vi "Measure P2.vi"(0 "Image Dup In":T1, 11 "Error In":errorcluster) -> (4 "Image Out":T1, 12 "Calibrated Results (P2 Hole)":sgl, 13 "Calibrated Results (P2 Left Edge Angles)":sgl, 14 "Calibrated Results (P2 Right Edge Angle)":sgl, 15 "Error Out":errorcluster)   [LabVIEW 2020, in "BilGör.lvlib"]
uses:
  <vilib>/vision/Image Controls.llb/IMAQ Image.ctl
  <vilib>/vision/Image Controls.llb/Vision Info Type2.ctl
  <vilib>/vision/Measure.llb/Edge Options.ctl
  <vilib>/vision/Measure.llb/Edge Polarity.ctl
  <vilib>/vision/Measure.llb/Straight Edge Options.ctl
  <vilib>/vision/Measure.llb/Straight Edge Process.ctl
  <vilib>/vision/NI_Vision_Development_Module.lvlib
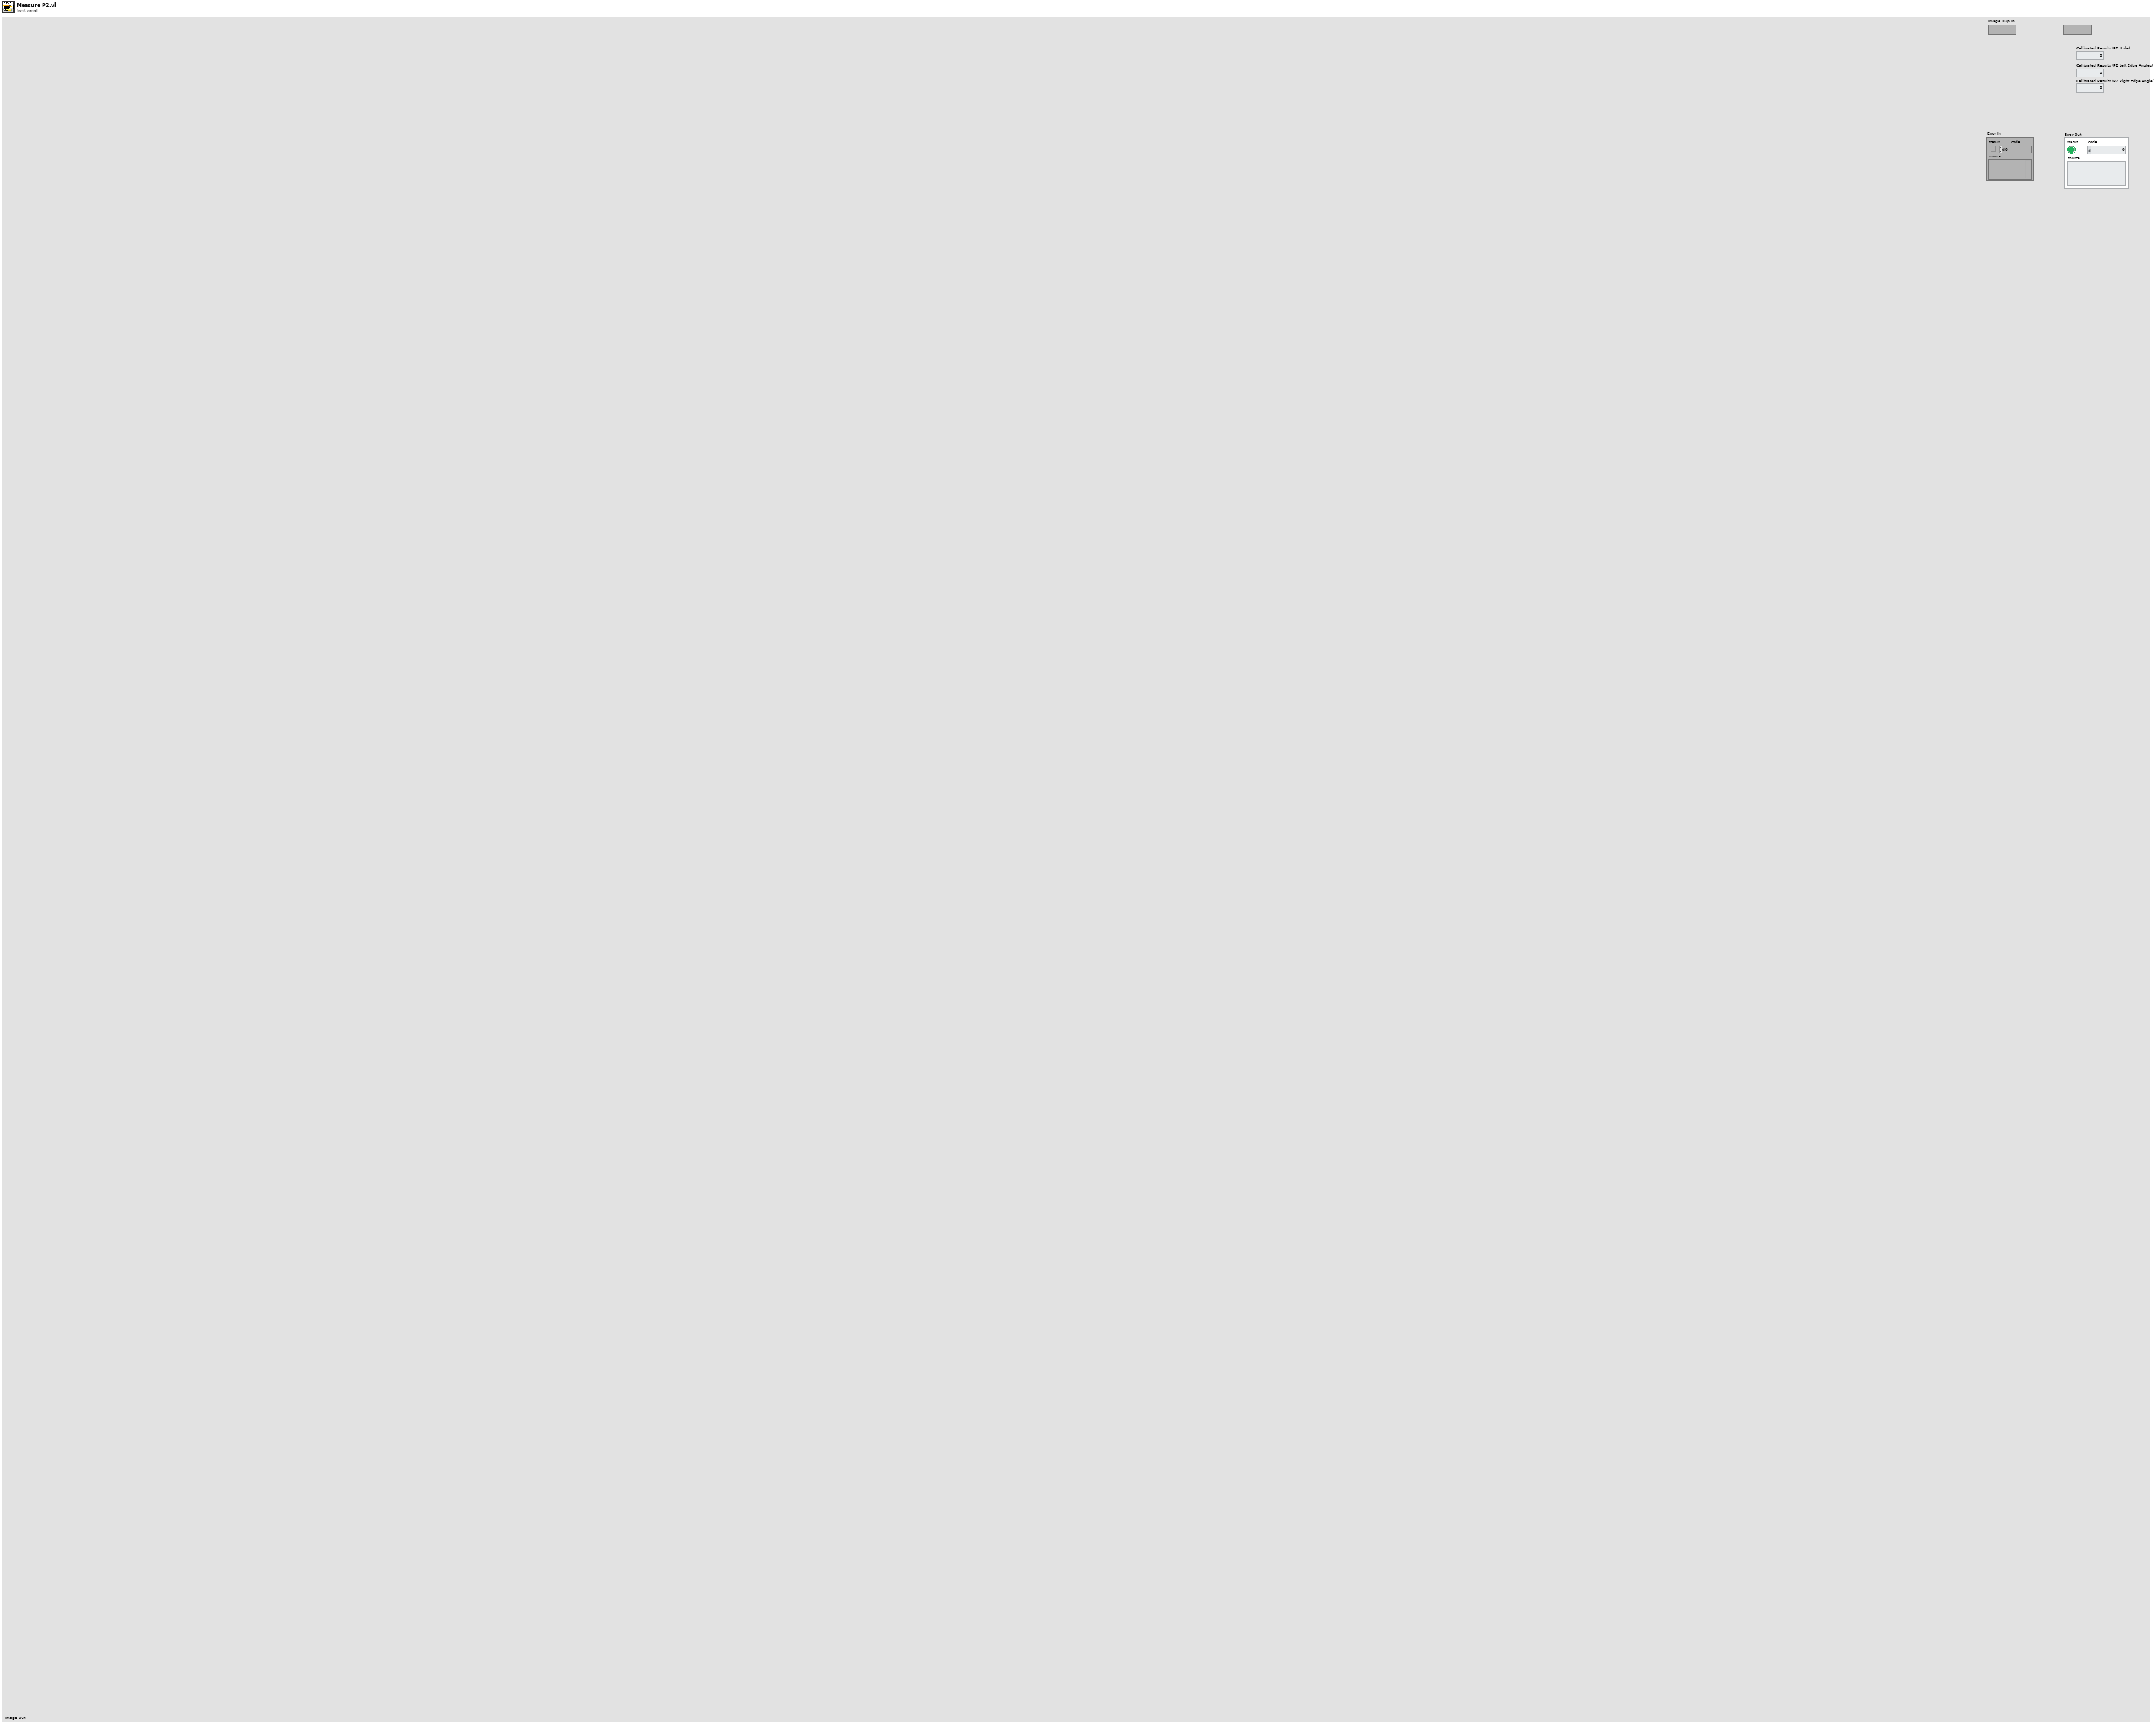
[diagram p1: front panel]
types:
  T1 = typedef "IMAQ Image.ctl" = refnum<image>
  T2 = cluster{"Origin":cluster{"X":sgl, "Y":sgl}, "Angle (deg)":sgl, "Axis Reference":u32}
  T3 = typedef "Straight Edge Options.ctl" = cluster{"Number of Lines":i32, "Type":T4, "Min. Score":dbl, "Max. Score":dbl, "Orientation":dbl, "Angle Range":dbl, "Angle Tolerance":dbl, "Step Size":u32, "Min. SNR (db)":dbl, "Min. Points (%)":dbl, "Hough Iterations":i32}
  T4 = typedef "Straight Edge Process.ctl" = enum32{"First Edge Rake", "Best Edge Rake", "Hough Edge Rake", "First Edge Projection", "Best Edge Projection"}
  T5 = typedef "Edge Options.ctl" = cluster{"Edge Polarity":T6, "Kernel Size":u32, "Width":u32, "Minimum Edge Strength":sgl, "Interpolation Type":enum32{"Zero Order", "Bilinear", "Quadratic", "Cubic", "Bilinear Fixed"}, "Data Processing Method":enum32{"Average", "Median"}}
  T6 = typedef "Edge Polarity.ctl" = u32
  T7 = cluster{"Search Direction":u32, "Edge Options":T5, "Show Search Area":bool, "Show Search Lines":bool, "Show Edges Found":bool, "Show Result":bool, "Search Area Color":u32, "Search Lines Color":u32, "Edge Locations Color":u32, "Result Color":u32, "Overlay Group Name":string}
  T8 = cluster{"Origin Pixel":cluster{"X":sgl, "Y":sgl}, "X Axis Pixel":cluster{"X":sgl, "Y":sgl}, "Axis Reference":u32}
  T9 = typedef "Simple Grid Descriptor" = cluster{"X Step":sgl, "Y Step":sgl, "Unit":T10}
  T10 = typedef "Image Unit" = enum32{"Undefined", "Angström", "Micrometer", "Millimeter", "Centimeter", "Meter", "Kilometer", "Microinch", "Inch", "Feet", "Nautical miles", "Standard miles", "Steps"}
  T11 = cluster{"Feature":u32, "Points IDs":cluster{"GUID":string, "Index":i32}[]}[]
  T12 = cluster{"Global Rectangle":i32[], "Contours":cluster{"ID":enum32{"External", "Internal"}, "Type":u32, "Coordinates":i32[]}[]}
  T13 = enum16{"Reset", "Update Coordinate System", "Get Coordinate System"}
  T14 = cluster{"Search  Direction":u32, "Edge Options":T5, "Show Search Area":bool, "Show Search Lines":bool, "Show Edges Found":bool, "Show Result":bool, "Search Area Color":u32, "Search Lines Color":u32, "Edge Locations Color":u32, "Result Color":u32, "Overlay Group Name":string}
  T15 = cluster{"Process":enum16{"Get First Edge", "Get First + Last Edge", "Get All Edges", "Get Best Edge"}, "Step Size":i32, "Max Pixel Radius":i32}
  T16 = typedef "Vision Info Type2.ctl" = u32
  T17 = typedef "IMAQ Coordinate System" = cluster{"Reference System":cluster{"Origin":cluster{"X":sgl, "Y":sgl}, "Angle (deg)":sgl, "Axis Reference":u32}, "Measurement System":cluster{"Origin":cluster{"X":sgl, "Y":sgl}, "Angle (deg)":sgl, "Axis Reference":u32}}
  T18 = typedef "ROI Descriptor" = cluster{"Global Rectangle":i32[], "Contours":cluster{"ID":enum32{"External", "Internal"}, "Type":u32, "Coordinates":i32[]}[]}
  T19 = cluster{"Point1 (Pixels)":cluster{"X":sgl, "Y":sgl}, "Point2 (Pixels)":cluster{"X":sgl, "Y":sgl}, "Point1 (Real-World)":cluster{"X":sgl, "Y":sgl}, "Point2 (Real-World)":cluster{"X":sgl, "Y":sgl}, "Angle (Pixel)":dbl, "Angle (Real-World)":dbl, "Score":dbl, "Straightness":dbl, "Average SNR (db)":dbl, "Calibration Valid":bool}[]
  T20 = cluster{"Center (Pixels)":cluster{"X":sgl, "Y":sgl}, "Radius (Pixels)":dbl, "Center (Real-World)":cluster{"X":sgl, "Y":sgl}, "Radius (Real-World)":dbl, "Roundness (Real-World)":dbl, "Average Strength":dbl, "Average SNR (dB)":dbl}
  T21 = cluster{"Point1 (Pixels)":cluster{"X":sgl, "Y":sgl}, "Point2 (Pixels)":cluster{"X":sgl, "Y":sgl}, "Point1 (Real-World)":cluster{"X":sgl, "Y":sgl}, "Point2 (Real-World)":cluster{"X":sgl, "Y":sgl}, "Angle (Pixel)":dbl, "Angle (Real-World)":dbl, "Score":dbl, "Straightness":dbl, "Average SNR (db)":dbl, "Calibration Valid":bool}
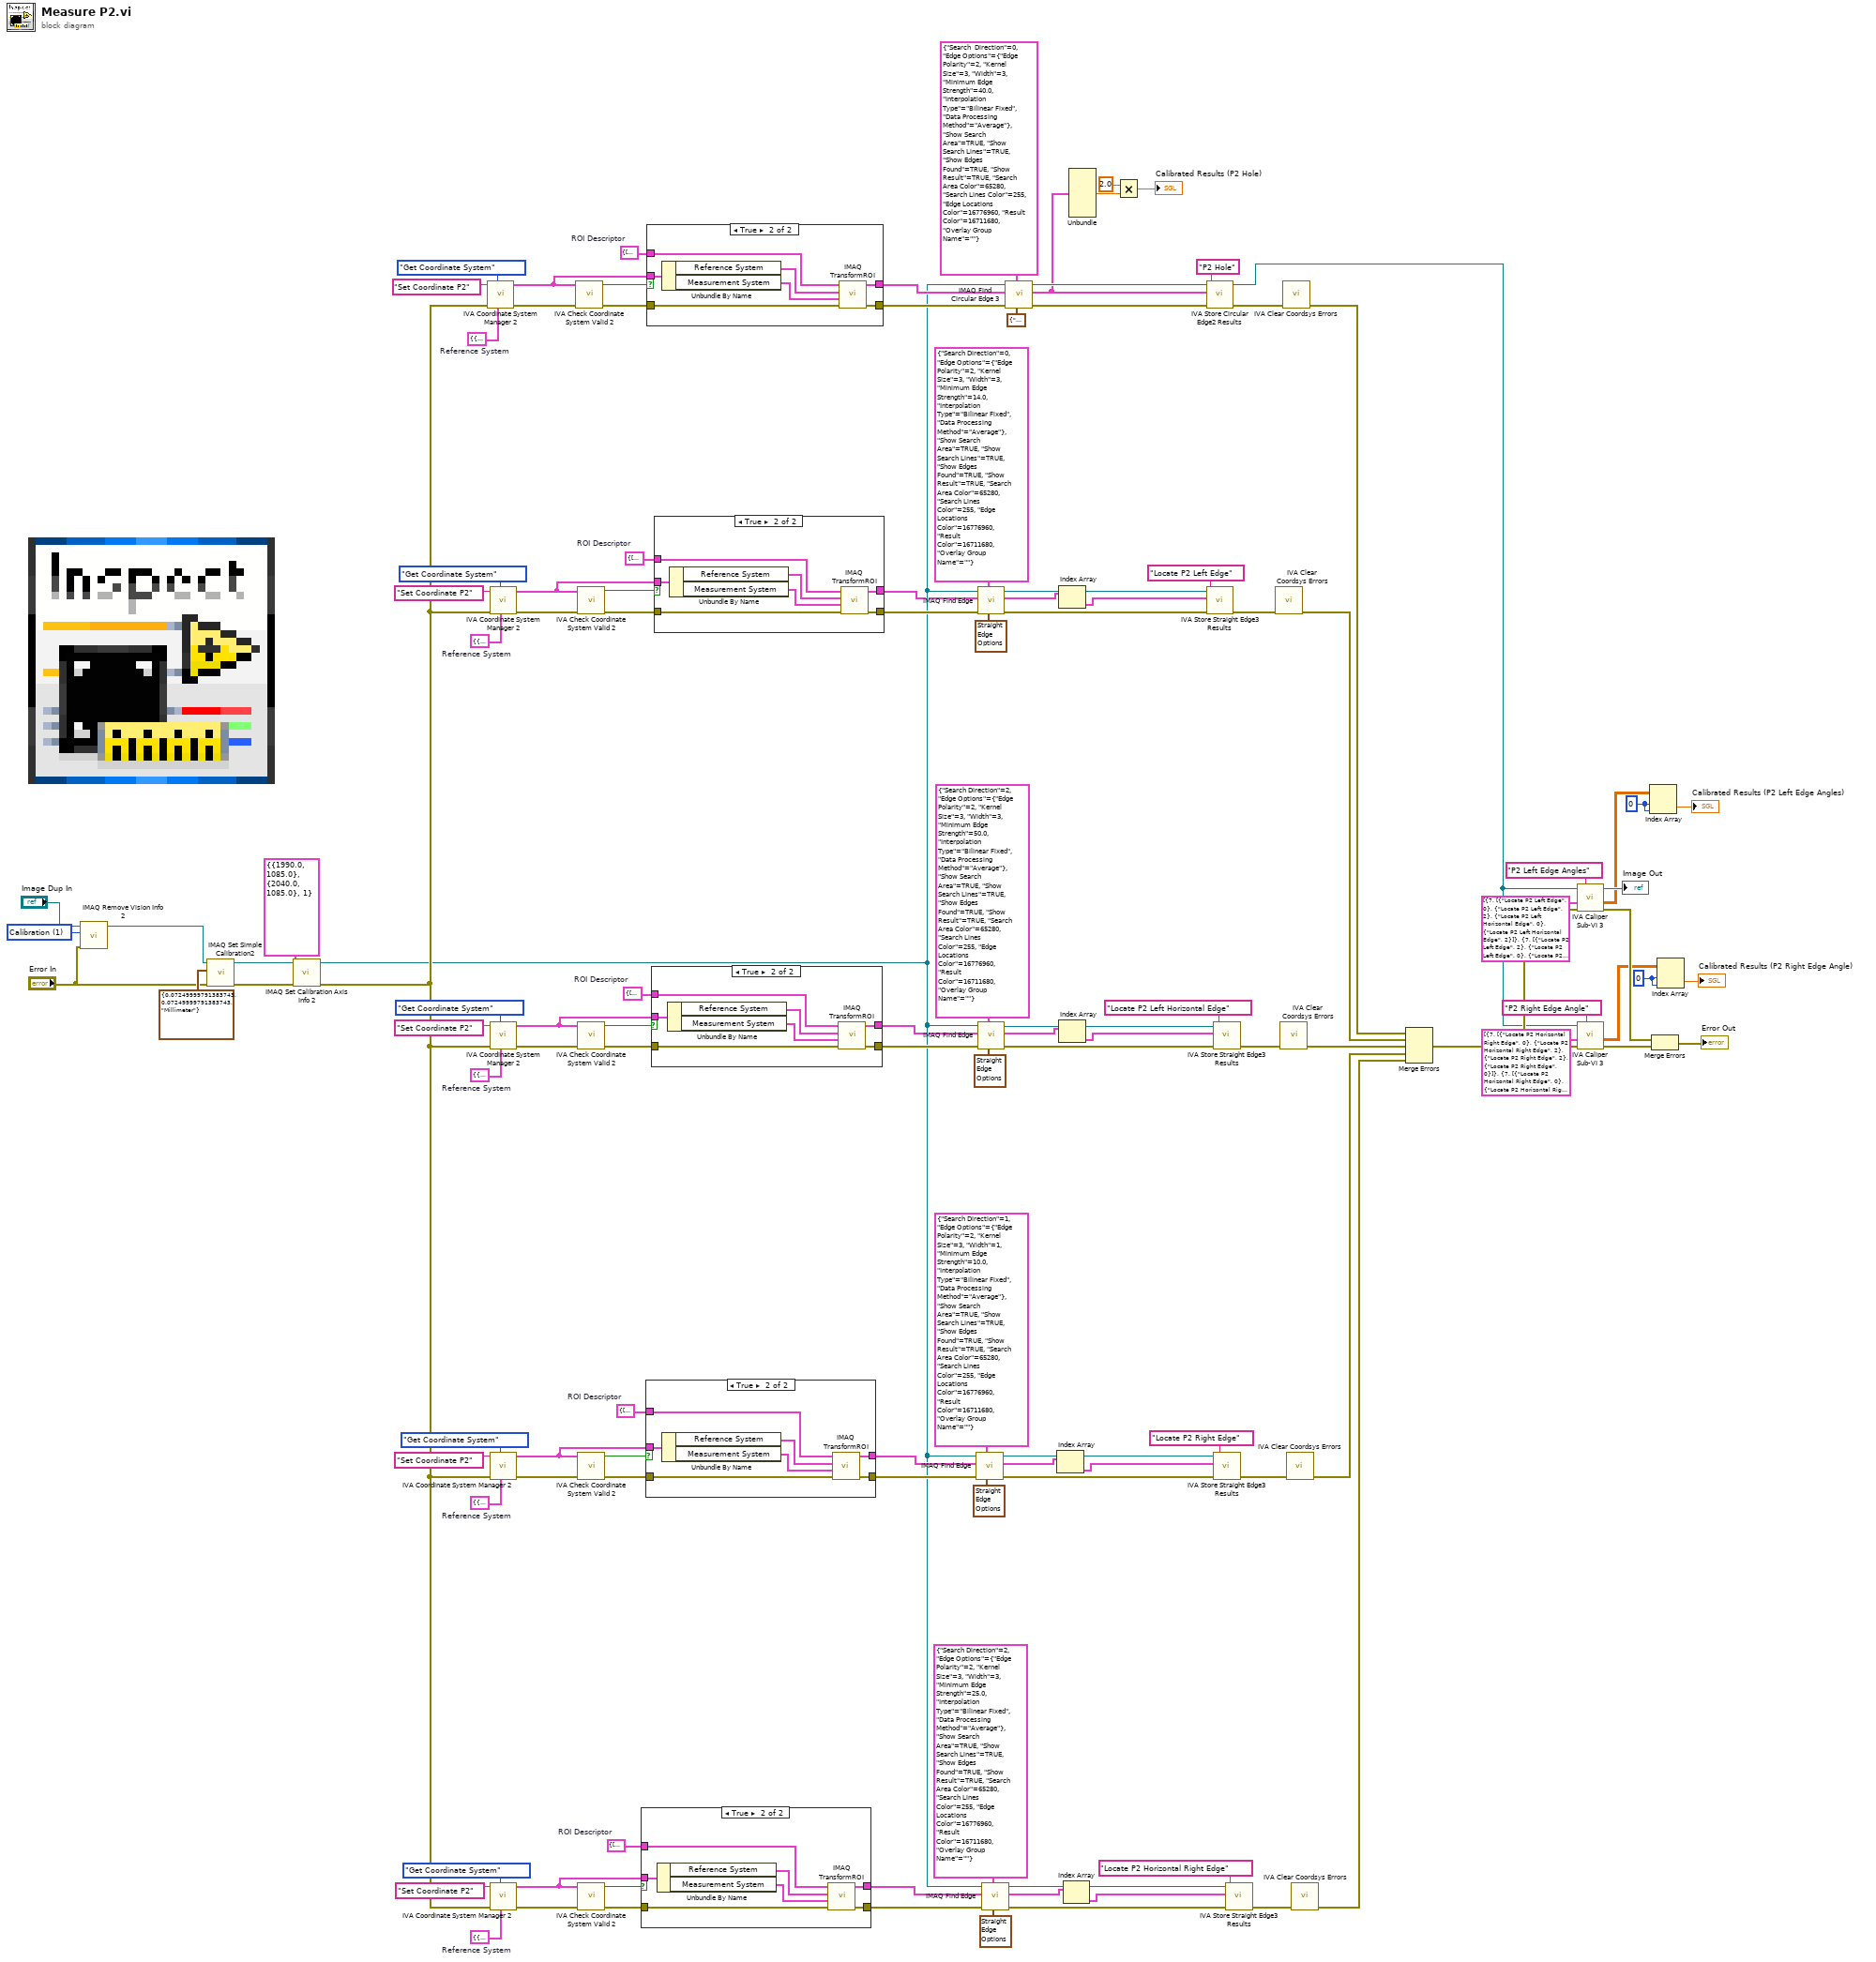
[diagram p0: block diagram]
diagram:
  w3 = 0 ("index (row)")
  w5 = 0 ("index (row)")
  w68 = T2 {"Origin"={"X"=2157.2554, "Y"=1094.1909}, "Angle (deg)"=0.0, "Axis Reference"=0}  # Reference System
  w48 = T12 {"Global Rectangle"=[2305, 827, 2590, 1102], "Contours"=[{"ID"=enum."External", "Type"=12, "Coordinates"=[2305, 827, 2590, 1102, 0]}]}  # ROI Descriptor
  w49 = T2 {"Origin"={"X"=2091.9243, "Y"=1142.8302}, "Angle (deg)"=0.0, "Axis Reference"=0}  # Reference System
  w67 = T12 {"Global Rectangle"=[2233, 374, 2483, 755], "Contours"=[{"ID"=enum."External", "Type"=12, "Coordinates"=[2233, 374, 2483, 755, 0]}]}  # ROI Descriptor
  w84 = T12 {"Global Rectangle"=[1389, 887, 1708, 1045], "Contours"=[{"ID"=enum."External", "Type"=12, "Coordinates"=[1389, 887, 1708, 1045, 0]}]}  # ROI Descriptor
  w85 = T2 {"Origin"={"X"=2157.2554, "Y"=1094.1909}, "Angle (deg)"=0.0, "Axis Reference"=0}  # Reference System
  w100 = T12 {"Global Rectangle"=[1545, 441, 1957, 867], "Contours"=[{"ID"=enum."External", "Type"=12, "Coordinates"=[1545, 441, 1957, 867, 0]}]}  # ROI Descriptor
  w101 = T2 {"Origin"={"X"=2157.2554, "Y"=1094.1909}, "Angle (deg)"=0.0, "Axis Reference"=0}  # Reference System
  w115 = T12 {"Global Rectangle"=[1957, 954, 2225, 1221], "Contours"=[{"ID"=enum."External", "Type"=7, "Coordinates"=[2090, 1087, 59, 133, 0, 0]}]}  # ROI Descriptor
  w116 = T2 {"Origin"={"X"=2091.9944, "Y"=1085.0201}, "Angle (deg)"=0.0, "Axis Reference"=0}  # Reference System
  w17 = T16 1 items=["Any", "Calibration", "Overlay", "Grayscale Template", "Color Template", "Geometric Template", "Custom Data", "Golden Template", "Geometric Template 2", "Contour Data", "Camera Model"] ("Vision Info")
  n1 = call "IMAQ Remove Vision Info 2"("error in (no error)"="Error In", "Vision Info"=w17, "Image"="Image Dup In") -> ("Image Out"=w122:T1)  [unwired: 8 out]
  n2 = call "IMAQ Set Simple Calibration2"("error in (no error)"="Error In", "Pixel Distances"=T9 {"X Step"=0.0725, "Y Step"=0.0725, "Unit"=enum."Millimeter"} ("Grid Descriptor"), "Image"=w122) -> ("error out"=w120:errorcluster, "Calibration Template Image"=w121:T1)  [unwired: 2 in, 5 out]
  n3 = call-poly "IMAQ Set Calibration Axis Info 2"("error in (no error)"=w120, "Calibration Axis Info"=T8 {"Origin Pixel"={"X"=1990.0, "Y"=1085.0}, "X Axis Pixel"={"X"=2040.0, "Y"=1085.0}, "Axis Reference"=1}, "Calibration Template Image In"=w121) -> ("error out"=w50:errorcluster, "Calibration Template Image Out"=w43:T1)  [unwired: 7 out]
  n4 = call <vilib>:"IVA Coordinate System Manager 2.vi"("Reference System"=w116, "Function"=T13."Get Coordinate System", "error in (no error)"=w50, "Coordinate System Name"="Set Coordinate P2") -> ("error out"=w112:errorcluster, "Coordinate System Out"=w114:T17)  [unwired: 3 in, 3 out]
  n5 = call <vilib>:"IVA Coordinate System Manager 2.vi"("Reference System"=w101, "Function"=T13."Get Coordinate System", "error in (no error)"=w50, "Coordinate System Name"="Set Coordinate P2") -> ("error out"=w98:errorcluster, "Coordinate System Out"=w16:T17)  [unwired: 3 in, 3 out]
  n6 = call <vilib>:"IVA Coordinate System Manager 2.vi"("Reference System"=w85, "Function"=T13."Get Coordinate System", "error in (no error)"=w50, "Coordinate System Name"="Set Coordinate P2") -> ("error out"=w81:errorcluster, "Coordinate System Out"=w83:T17)  [unwired: 3 in, 3 out]
  n7 = call <vilib>:"IVA Coordinate System Manager 2.vi"("Reference System"=w68, "Function"=T13."Get Coordinate System", "error in (no error)"=w50, "Coordinate System Name"="Set Coordinate P2") -> ("error out"=w64:errorcluster, "Coordinate System Out"=w66:T17)  [unwired: 3 in, 3 out]
  n8 = call <vilib>:"IVA Coordinate System Manager 2.vi"("Reference System"=w49, "Function"=T13."Get Coordinate System", "error in (no error)"=w50, "Coordinate System Name"="Set Coordinate P2") -> ("error out"=w45:errorcluster, "Coordinate System Out"=w47:T17)  [unwired: 3 in, 3 out]
  n9 = call <vilib>:"IVA Check Coordinate System Valid 2.vi"("error in (no error)"=w112, "Coordinate System"=w114) -> ("error out"=w111:errorcluster, "Valid?"=w113:bool)  [unwired: 8 out]
  n10 = call <vilib>:"IVA Check Coordinate System Valid 2.vi"("error in (no error)"=w98, "Coordinate System"=w16) -> ("error out"=w97:errorcluster, "Valid?"=w99:bool)  [unwired: 8 out]
  n11 = call <vilib>:"IVA Check Coordinate System Valid 2.vi"("error in (no error)"=w81, "Coordinate System"=w83) -> ("error out"=w80:errorcluster, "Valid?"=w82:bool)  [unwired: 8 out]
  n12 = call <vilib>:"IVA Check Coordinate System Valid 2.vi"("error in (no error)"=w64, "Coordinate System"=w66) -> ("error out"=w63:errorcluster, "Valid?"=w65:bool)  [unwired: 8 out]
  n13 = call <vilib>:"IVA Check Coordinate System Valid 2.vi"("error in (no error)"=w45, "Coordinate System"=w47) -> ("error out"=w44:errorcluster, "Valid?"=w46:bool)  [unwired: 8 out]
  n14 = case shown="True" w46 {
    tunnel: w48 -> [w125 w132]
    tunnel: [w125 w129] -> w42
    tunnel: [w124 w128] -> w40
    tunnel: w47 -> [_ w127]
    tunnel: w44 -> [w124 w126]
    frame False {
    }
    frame True {
      n15 = Unbundle By Name(w127) -> ("Reference System"=w131:T2, "Measurement System"=w130:T2)
      n16 = call "IMAQ TransformROI"("error in (no error)"=w126, "New Reference"=w130, "Base Reference"=w131, "ROI Descriptor"=w132) -> ("error out"=w128:errorcluster, "ROI Descriptor out"=w129:T18)  [unwired: 6 out]
    }
  }
  n17 = case shown="True" w65 {
    tunnel: w67 -> [w134 w141]
    tunnel: [w134 w138] -> w62
    tunnel: [w133 w137] -> w60
    tunnel: w66 -> [_ w136]
    tunnel: w63 -> [w133 w135]
    frame False {
    }
    frame True {
      n18 = Unbundle By Name(w136) -> ("Reference System"=w140:T2, "Measurement System"=w139:T2)
      n19 = call "IMAQ TransformROI"("error in (no error)"=w135, "New Reference"=w139, "Base Reference"=w140, "ROI Descriptor"=w141) -> ("error out"=w137:errorcluster, "ROI Descriptor out"=w138:T18)  [unwired: 6 out]
    }
  }
  n20 = case shown="True" w113 {
    tunnel: w115 -> [w143 w150]
    tunnel: [w143 w147] -> w109
    tunnel: [w142 w146] -> w108
    tunnel: w114 -> [_ w145]
    tunnel: w111 -> [w142 w144]
    frame False {
    }
    frame True {
      n21 = Unbundle By Name(w145) -> ("Reference System"=w149:T2, "Measurement System"=w148:T2)
      n22 = call "IMAQ TransformROI"("error in (no error)"=w144, "New Reference"=w148, "Base Reference"=w149, "ROI Descriptor"=w150) -> ("error out"=w146:errorcluster, "ROI Descriptor out"=w147:T18)  [unwired: 6 out]
    }
  }
  n23 = case shown="True" w82 {
    tunnel: w84 -> [w152 w159]
    tunnel: [w152 w156] -> w15
    tunnel: [w151 w155] -> w78
    tunnel: w83 -> [_ w154]
    tunnel: w80 -> [w151 w153]
    frame False {
    }
    frame True {
      n24 = Unbundle By Name(w154) -> ("Reference System"=w158:T2, "Measurement System"=w157:T2)
      n25 = call "IMAQ TransformROI"("error in (no error)"=w153, "New Reference"=w157, "Base Reference"=w158, "ROI Descriptor"=w159) -> ("error out"=w155:errorcluster, "ROI Descriptor out"=w156:T18)  [unwired: 6 out]
    }
  }
  n26 = case shown="True" w99 {
    tunnel: w100 -> [w161 w168]
    tunnel: [w161 w165] -> w14
    tunnel: [w160 w164] -> w95
    tunnel: w16 -> [_ w163]
    tunnel: w97 -> [w160 w162]
    frame False {
    }
    frame True {
      n27 = Unbundle By Name(w163) -> ("Reference System"=w167:T2, "Measurement System"=w166:T2)
      n28 = call "IMAQ TransformROI"("error in (no error)"=w162, "New Reference"=w166, "Base Reference"=w167, "ROI Descriptor"=w168) -> ("error out"=w164:errorcluster, "ROI Descriptor out"=w165:T18)  [unwired: 6 out]
    }
  }
  n29 = call "IMAQ Find Edge"("Line Fit Options"=T3 {"Number of Lines"=1, "Type"=enum."First Edge Rake", "Min. Score"=10.0, "Max. Score"=1000.0, "Orientation"=0.0, "Angle Range"=45.0, "Angle Tolerance"=1.0, "Step Size"=38, "Min. SNR (db)"=0.0, "Min. Points (%)"=25.0, "Hough Iterations"=5} ("Fit Options"), "Options"=T7 {"Search Direction"=1, "Edge Options"={"Edge Polarity"=2, "Kernel Size"=3, "Width"=1, "Minimum Edge Strength"=10.0, "Interpolation Type"=enum."Bilinear Fixed", "Data Processing Method"=enum."Average"}, "Show Search Area"=TRUE, "Show Search Lines"=TRUE, "Show Edges Found"=TRUE, "Show Result"=TRUE, "Search Area Color"=65280, "Search Lines Color"=255, "Edge Locations Color"=16776960, "Result Color"=16711680, "Overlay Group Name"=""}, "error in (no error)"=w60, "ROI Descriptor"=w62, "Image"=w43) -> ("error out"=w55:errorcluster, "Straight Edges"=w54:T19, "Image Out"=w56:T1)  [unwired: 1 in, 3 out]
  n30 = call "IMAQ Find Edge"("Line Fit Options"=T3 {"Number of Lines"=1, "Type"=enum."First Edge Rake", "Min. Score"=10.0, "Max. Score"=1000.0, "Orientation"=0.0, "Angle Range"=45.0, "Angle Tolerance"=1.0, "Step Size"=43, "Min. SNR (db)"=0.0, "Min. Points (%)"=25.0, "Hough Iterations"=5} ("Fit Options"), "Options"=T7 {"Search Direction"=0, "Edge Options"={"Edge Polarity"=2, "Kernel Size"=3, "Width"=3, "Minimum Edge Strength"=14.0, "Interpolation Type"=enum."Bilinear Fixed", "Data Processing Method"=enum."Average"}, "Show Search Area"=TRUE, "Show Search Lines"=TRUE, "Show Edges Found"=TRUE, "Show Result"=TRUE, "Search Area Color"=65280, "Search Lines Color"=255, "Edge Locations Color"=16776960, "Result Color"=16711680, "Overlay Group Name"=""}, "error in (no error)"=w95, "ROI Descriptor"=w14, "Image"=w43) -> ("error out"=w90:errorcluster, "Straight Edges"=w89:T19, "Image Out"=w91:T1)  [unwired: 1 in, 3 out]
  n31 = call "IMAQ Find Edge"("Line Fit Options"=T3 {"Number of Lines"=1, "Type"=enum."First Edge Rake", "Min. Score"=10.0, "Max. Score"=1000.0, "Orientation"=0.0, "Angle Range"=45.0, "Angle Tolerance"=1.0, "Step Size"=32, "Min. SNR (db)"=0.0, "Min. Points (%)"=25.0, "Hough Iterations"=5} ("Fit Options"), "Options"=T7 {"Search Direction"=2, "Edge Options"={"Edge Polarity"=2, "Kernel Size"=3, "Width"=3, "Minimum Edge Strength"=50.0, "Interpolation Type"=enum."Bilinear Fixed", "Data Processing Method"=enum."Average"}, "Show Search Area"=TRUE, "Show Search Lines"=TRUE, "Show Edges Found"=TRUE, "Show Result"=TRUE, "Search Area Color"=65280, "Search Lines Color"=255, "Edge Locations Color"=16776960, "Result Color"=16711680, "Overlay Group Name"=""}, "error in (no error)"=w78, "ROI Descriptor"=w15, "Image"=w43) -> ("error out"=w73:errorcluster, "Straight Edges"=w72:T19, "Image Out"=w74:T1)  [unwired: 1 in, 3 out]
  n32 = call "IMAQ Find Edge"("Line Fit Options"=T3 {"Number of Lines"=1, "Type"=enum."First Edge Rake", "Min. Score"=10.0, "Max. Score"=1000.0, "Orientation"=0.0, "Angle Range"=45.0, "Angle Tolerance"=1.0, "Step Size"=28, "Min. SNR (db)"=0.0, "Min. Points (%)"=25.0, "Hough Iterations"=5} ("Fit Options"), "Options"=T7 {"Search Direction"=2, "Edge Options"={"Edge Polarity"=2, "Kernel Size"=3, "Width"=3, "Minimum Edge Strength"=25.0, "Interpolation Type"=enum."Bilinear Fixed", "Data Processing Method"=enum."Average"}, "Show Search Area"=TRUE, "Show Search Lines"=TRUE, "Show Edges Found"=TRUE, "Show Result"=TRUE, "Search Area Color"=65280, "Search Lines Color"=255, "Edge Locations Color"=16776960, "Result Color"=16711680, "Overlay Group Name"=""}, "error in (no error)"=w40, "ROI Descriptor"=w42, "Image"=w43) -> ("error out"=w35:errorcluster, "Straight Edges"=w34:T19, "Image Out"=w36:T1)  [unwired: 1 in, 3 out]
  n33 = call "IMAQ Find Circular Edge 3"("Circle Fit Options"=T15 {"Process"=enum."Get Best Edge", "Step Size"=10, "Max Pixel Radius"=3}, "Options"=T14 {"Search  Direction"=0, "Edge Options"={"Edge Polarity"=2, "Kernel Size"=3, "Width"=3, "Minimum Edge Strength"=40.0, "Interpolation Type"=enum."Bilinear Fixed", "Data Processing Method"=enum."Average"}, "Show Search Area"=TRUE, "Show Search Lines"=TRUE, "Show Edges Found"=TRUE, "Show Result"=TRUE, "Search Area Color"=65280, "Search Lines Color"=255, "Edge Locations Color"=16776960, "Result Color"=16711680, "Overlay Group Name"=""}, "error in (no error)"=w108, "ROI Descriptor"=w109, "Image"=w43) -> ("error out"=w13:errorcluster, "Fitted Circle"=w10:T20, "Image Out"=w105:T1)  [unwired: 2 in, 2 out]
  n34 = Index Array(array=w54) -> (element=w57:T21)  [unwired: 1 in]
  n35 = Index Array(array=w89) -> (element=w92:T21)  [unwired: 1 in]
  n36 = Index Array(array=w72) -> (element=w75:T21)  [unwired: 1 in]
  n37 = Index Array(array=w34) -> (element=w37:T21)  [unwired: 1 in]
  n38 = Unbundle(w10) -> ("Radius (Real-World)"=w9:dbl)  [unwired: 6 out]
  n39 = Multiply(x=2.0, y=w9) -> (x*y=→"Calibrated Results (P2 Hole)":dbl)
  n40 = call <vilib>:"IVA Store Circular Edge2 Results.vi"("error in (no error)"=w13, "Step Name"="P2 Hole", "Fitted Circle"=w10, "Image in"=w105) -> ("error out"=w104:errorcluster, "Image dup"=w12:T1)  [unwired: 2 in, 4 out]
  n41 = call <vilib>:"IVA Store Straight Edge3 Results.vi"("error in (no error)"=w90, "Step Name"="Locate P2 Left Edge", "Straight Edge"=w92, "Image in"=w91) -> ("error out"=w88:errorcluster)  [unwired: 1 in, 6 out]
  n42 = call <vilib>:"IVA Store Straight Edge3 Results.vi"("error in (no error)"=w73, "Step Name"="Locate P2 Left Horizontal Edge", "Straight Edge"=w75, "Image in"=w74) -> ("error out"=w71:errorcluster)  [unwired: 1 in, 6 out]
  n43 = call <vilib>:"IVA Store Straight Edge3 Results.vi"("error in (no error)"=w55, "Step Name"="Locate P2 Right Edge", "Straight Edge"=w57, "Image in"=w56) -> ("error out"=w53:errorcluster)  [unwired: 1 in, 6 out]
  n44 = call <vilib>:"IVA Store Straight Edge3 Results.vi"("error in (no error)"=w35, "Step Name"="Locate P2 Horizontal Right Edge", "Straight Edge"=w37, "Image in"=w36) -> ("error out"=w33:errorcluster)  [unwired: 1 in, 6 out]
  n45 = call <vilib>:"IVA Clear Coordsys Errors.vi"("error in (no error)"=w88) -> ("error out"=w31:errorcluster)  [unwired: 10 in]
  n46 = call <vilib>:"IVA Clear Coordsys Errors.vi"("error in (no error)"=w71) -> ("error out"=w30:errorcluster)  [unwired: 10 in]
  n47 = call <vilib>:"IVA Clear Coordsys Errors.vi"("error in (no error)"=w104) -> ("error out"=w32:errorcluster)  [unwired: 10 in]
  n48 = call <vilib>:"IVA Clear Coordsys Errors.vi"("error in (no error)"=w53) -> ("error out"=w29:errorcluster)  [unwired: 10 in]
  n49 = call <vilib>:"IVA Clear Coordsys Errors.vi"("error in (no error)"=w33) -> ("error out"=w28:errorcluster)  [unwired: 10 in]
  n50 = Merge Errors(w32, w31, w30, w29, w28) -> (w25:errorcluster)
  n51 = call <vilib>:"IVA Caliper Sub-VI 3.vi"("error in"=w25, "Parameters"=T11 [{"Feature"=7, "Points IDs"=[{"GUID"="Locate P2 Left Edge", "Index"=0}, {"GUID"="Locate P2 Left Edge", "Index"=2}, {"GUID"="Locate P2 Left Horizontal Edge", "Index"=0}, {"GUID"="Locate P2 Left Horizontal Edge", "Index"=2}]}, {"Feature"=7, "Points IDs"=[{"GUID"="Locate P2 Left Edge", "Index"=2}, {"GUID"="Locate P2 Left Edge", "Index"=0}, {"GUID"="Locate P2 Left Horizontal Edge", "Index"=2}, {"GUID"="Locate P2 Left Horizontal Edge", "Index"=0}]}, {"Feature"=7, "Points IDs"=[{"GUID"="Locate P2 Left Edge", "Index"=0}, {"GUID"="Locate P2 Left Edge", "Index"=2}, {"GUID"="Locate P2 Left Horizontal Edge", "Index"=0}, {"GUID"="Locate P2 Left Horizontal Edge", "Index"=2}]}], "Step Name"="P2 Left Edge Angles", "Image In"=w12) -> ("error out"=w20:errorcluster, "Results (Calibrated)"=w6:sgl[][], "Image Out"=→"Image Out":T1)  [unwired: 1 in, 4 out]
  n52 = call <vilib>:"IVA Caliper Sub-VI 3.vi"("error in"=w25, "Parameters"=T11 [{"Feature"=7, "Points IDs"=[{"GUID"="Locate P2 Horizontal Right Edge", "Index"=0}, {"GUID"="Locate P2 Horizontal Right Edge", "Index"=2}, {"GUID"="Locate P2 Right Edge", "Index"=2}, {"GUID"="Locate P2 Right Edge", "Index"=0}]}, {"Feature"=7, "Points IDs"=[{"GUID"="Locate P2 Horizontal Right Edge", "Index"=0}, {"GUID"="Locate P2 Horizontal Right Edge", "Index"=2}, {"GUID"="Locate P2 Right Edge", "Index"=2}, {"GUID"="Locate P2 Right Edge", "Index"=0}]}, {"Feature"=7, "Points IDs"=[{"GUID"="Locate P2 Horizontal Right Edge", "Index"=0}, {"GUID"="Locate P2 Horizontal Right Edge", "Index"=2}, {"GUID"="Locate P2 Right Edge", "Index"=2}, {"GUID"="Locate P2 Right Edge", "Index"=0}]}, {"Feature"=7, "Points IDs"=[{"GUID"="Locate P2 Horizontal Right Edge", "Index"=0}, {"GUID"="Locate P2 Horizontal Right Edge", "Index"=2}, {"GUID"="Locate P2 Right Edge", "Index"=2}, {"GUID"="Locate P2 Right Edge", "Index"=0}]}, {"Feature"=7, "Points IDs"=[{"GUID"="Locate P2 Horizontal Right Edge", "Index"=0}, {"GUID"="Locate P2 Horizontal Right Edge", "Index"=2}, {"GUID"="Locate P2 Right Edge", "Index"=2}, {"GUID"="Locate P2 Right Edge", "Index"=0}]}, {"Feature"=7, "Points IDs"=[{"GUID"="Locate P2 Horizontal Right Edge", "Index"=0}, {"GUID"="Locate P2 Horizontal Right Edge", "Index"=2}, {"GUID"="Locate P2 Right Edge", "Index"=2}, {"GUID"="Locate P2 Right Edge", "Index"=0}]}, {"Feature"=7, "Points IDs"=[{"GUID"="Locate P2 Horizontal Right Edge", "Index"=0}, {"GUID"="Locate P2 Horizontal Right Edge", "Index"=2}, {"GUID"="Locate P2 Right Edge", "Index"=2}, {"GUID"="Locate P2 Right Edge", "Index"=0}]}, {"Feature"=7, "Points IDs"=[{"GUID"="Locate P2 Horizontal Right Edge", "Index"=0}, {"GUID"="Locate P2 Horizontal Right Edge", "Index"=2}, {"GUID"="Locate P2 Right Edge", "Index"=2}, {"GUID"="Locate P2 Right Edge", "Index"=0}]}], "Step Name"="P2 Right Edge Angle", "Image In"=w12) -> ("error out"=w19:errorcluster, "Results (Calibrated)"=w2:sgl[][])  [unwired: 1 in, 5 out]
  n53 = Index Array(array=w6, index (row)=w5, index (col)=w5) -> (element=→"Calibrated Results (P2 Left Edge Angles)":sgl)
  n54 = Merge Errors(w20, w19) -> (→"Error Out":errorcluster)
  n55 = Index Array(array=w2, index (row)=w3, index (col)=w3) -> (element=→"Calibrated Results (P2 Right Edge Angle)":sgl)
